vi "Begin.vi"(8 "error in":errorcluster) -> (0 "error out":errorcluster)   [LabVIEW 2017]
doc: "Called before other user functions, this VI is expected to open initial I/O refnums, load in file data, and do all program initialization. Notice that the <B>error out</B> terminal is simply used for data flow. Wiring it to other structures or subVIs ensures that this VI runs first."
uses:
  <vilib>/Rock Robotics/WPI/DriverStation/WPI_DriverStationRobotMode2.ctl
  <vilib>/Rock Robotics/WPI/Joystick/WPI_JoystickDeviceEnum.ctl
  <vilib>/Rock Robotics/WPI/Solenoid/WPI_SolenoidChannel.ctl
  <vilib>/Rock Robotics/SystemInterfaces/DIO/FPGA_DIOChannel.ctl
  <vilib>/Rock Robotics/SystemInterfaces/DIO/FPGA_DIOPWMChannel.ctl
  <vilib>/Rock Robotics/SystemInterfaces/spilib/spi_bus.ctl
  Robot Global Data.vi
  <vilib>/Rock Robotics/Network Tables/NT Write String Array.vi
  <vilib>/Rock Robotics/WPI/Solenoid/WPI_SolenoidOpenDouble.vi
  <vilib>/Rock Robotics/WPI/Ultrasonic/WPI_SonarMB1010DigitalOpen.vi
  <vilib>/Rock Robotics/WPI/Ultrasonic/WPI_SonarMB1010DigRefNum Registry Set.vi
  <vilib>/Rock Robotics/WPI/Switch/WPI_SwitchOpenLimit.vi
  <vilib>/Rock Robotics/WPI/MotorControl/WPI_MotorControlOpen VictorSP.vi
  <vilib>/Rock Robotics/WPI/Gyro/WPI_GyroXRS450_SPI_Open.vi
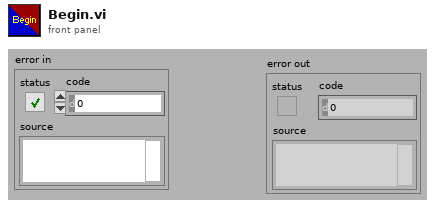
[diagram p1: front panel]
types:
  T1 = typedef "spi_bus.ctl" = enum16{"SPI On-Board, CS0", "SPI On-Board, CS1", "SPI On-Board, CS2", "SPI On-Board, CS3", "SPI MXP", "Invalid"}
  T2 = typedef "FPGA_DIOPWMChannel.ctl" = enum8{"PWM 0", "PWM 1", "PWM 2", "PWM 3", "PWM 4", "PWM 5", "PWM 6", "PWM 7", "PWM 8", "PWM 9", "PWM MXP 0", "PWM MXP 1", "PWM MXP 2", "PWM MXP 3", "PWM MXP 4", "PWM MXP 5", "PWM MXP 6", "PWM MXP 7", "PWM MXP 8", "PWM MXP 9", "Invalid"}
  T3 = typedef "FPGA_DIOChannel.ctl" = enum8{"DIO 0", "DIO 1", "DIO 2", "DIO 3", "DIO 4", "DIO 5", "DIO 6", "DIO 7", "DIO 8", "DIO 9", "DIO MXP 0", "DIO MXP 1", "DIO MXP 2", "DIO MXP 3", "DIO MXP 4", "DIO MXP 5", "DIO MXP 6", "DIO MXP 7", "DIO MXP 8", "DIO MXP 9", "DIO MXP 10", "DIO MXP 11", "DIO MXP 12", "DIO MXP 13", "DIO MXP 14", "DIO MXP 15", "SPI Port CS1", "SPI Port CS2", "SPI Port CS3", "SPI Port MISO", "SPI Port MOSI", "Invalid"}
  T4 = typedef "WPI_SolenoidChannel.ctl" = enum8{"Solenoid 0", "Solenoid 1", "Solenoid 2", "Solenoid 3", "Solenoid 4", "Solenoid 5", "Solenoid 6", "Solenoid 7", "Invalid"}
  T5 = typedef "WPI_JoystickDeviceEnum.ctl" = enum16{"USB 0", "USB 1", "USB 2", "USB 3", "USB 4", "USB 5"}
  T6 = typedef "WPI_DriverStationRobotMode2.ctl" = enum16{"Autonomous Disabled", "Autonomous Enabled", "Teleop Disabled", "Teleop Enabled", "Disconnected", "Finish", "Test Disabled", "Test Enabled", "Emergency Stopped"}
  T7 = typedef "WPI_MotorControlDeviceRef.ctl" = cluster{"DeviceStatus":errorcluster, "Type":T8, "PWM":cluster{"PWM Channel":T2, "DeadBand":T9}, "CAN":cluster{"Device Number":u8, "SetOutput VI Ref":variant, "GetOutput VI Ref":variant, "Enable VI Ref":variant, "Disable VI Ref":variant, "Data":variant}, "Invert":bool, "DIO PWM":cluster{"PWM \"Enable\" Channel":T2, "DIOChannel":T3, "PWM Rate":dbl}}
  T8 = typedef "WPI_MotorControlType.ctl" = enum16{"PWM", "CAN", "DIO PWM"}
  T9 = typedef "WPI_PWMDeadband.ctl" = cluster{"Name":string, "maxPositivePwm":i32, "minPositivePwm":i32, "centerPwm":i32, "maxNegativePwm":i32, "minNegativePwm":i32, "angularRange":u16}
  T10 = typedef "WPI_SwitchDevRef.ctl" = cluster{"DevStatus":errorcluster, "DIO Channel":T3, "CntIndex":T11, "Normally Closed":bool}
  T11 = typedef "FPGA_CounterCtrSystemIndex.ctl" = enum8{"Ctr 0", "Ctr 1", "Ctr 2", "Ctr 3", "Ctr 4", "Ctr 5", "Ctr 6", "Ctr 7", "Invalid"}
  T12 = typedef "WPI_SonarMB1010DigitalDeviceRef.ctl" = cluster{"CounterDevRef":T13, "Scaling factor (s/in)":dbl}
  T13 = typedef "WPI_CounterDevRef.ctl" = cluster{"DevStatus":errorcluster, "CntIndex":T11}
  T14 = typedef "WPI_GyroDevRef.ctl" = cluster{"DevStatus":errorcluster, "Analog Channel":T15, "Gain (VoltsPerDegree/Second)":dbl, "Gyro Type":enum16{"Analog", "XRS450"}, "Handle":i32, "SPI Bus":T1, "Device Found":bool, "Sample Rate":dbl, "Calibrate On Open":bool, "Offset":dbl}
  T15 = typedef "FPGA_AIChannel.ctl" = enum8{"AI 0", "AI 1", "AI 2", "AI 3", "AI MXP 0", "AI MXP 1", "AI MXP 2", "AI MXP 3", "Invalid"}
  T16 = typedef "WPI_SolenoidDevRef.ctl" = cluster{"DevStatus":errorcluster, "Pneumatics Control Module":u8, "Forward Solenoid Channel":T4, "Reverse Solenoid Channel":T4}
  T17 = typedef "WPI_JoystickDevRef.ctl" = cluster{"Device":T5}
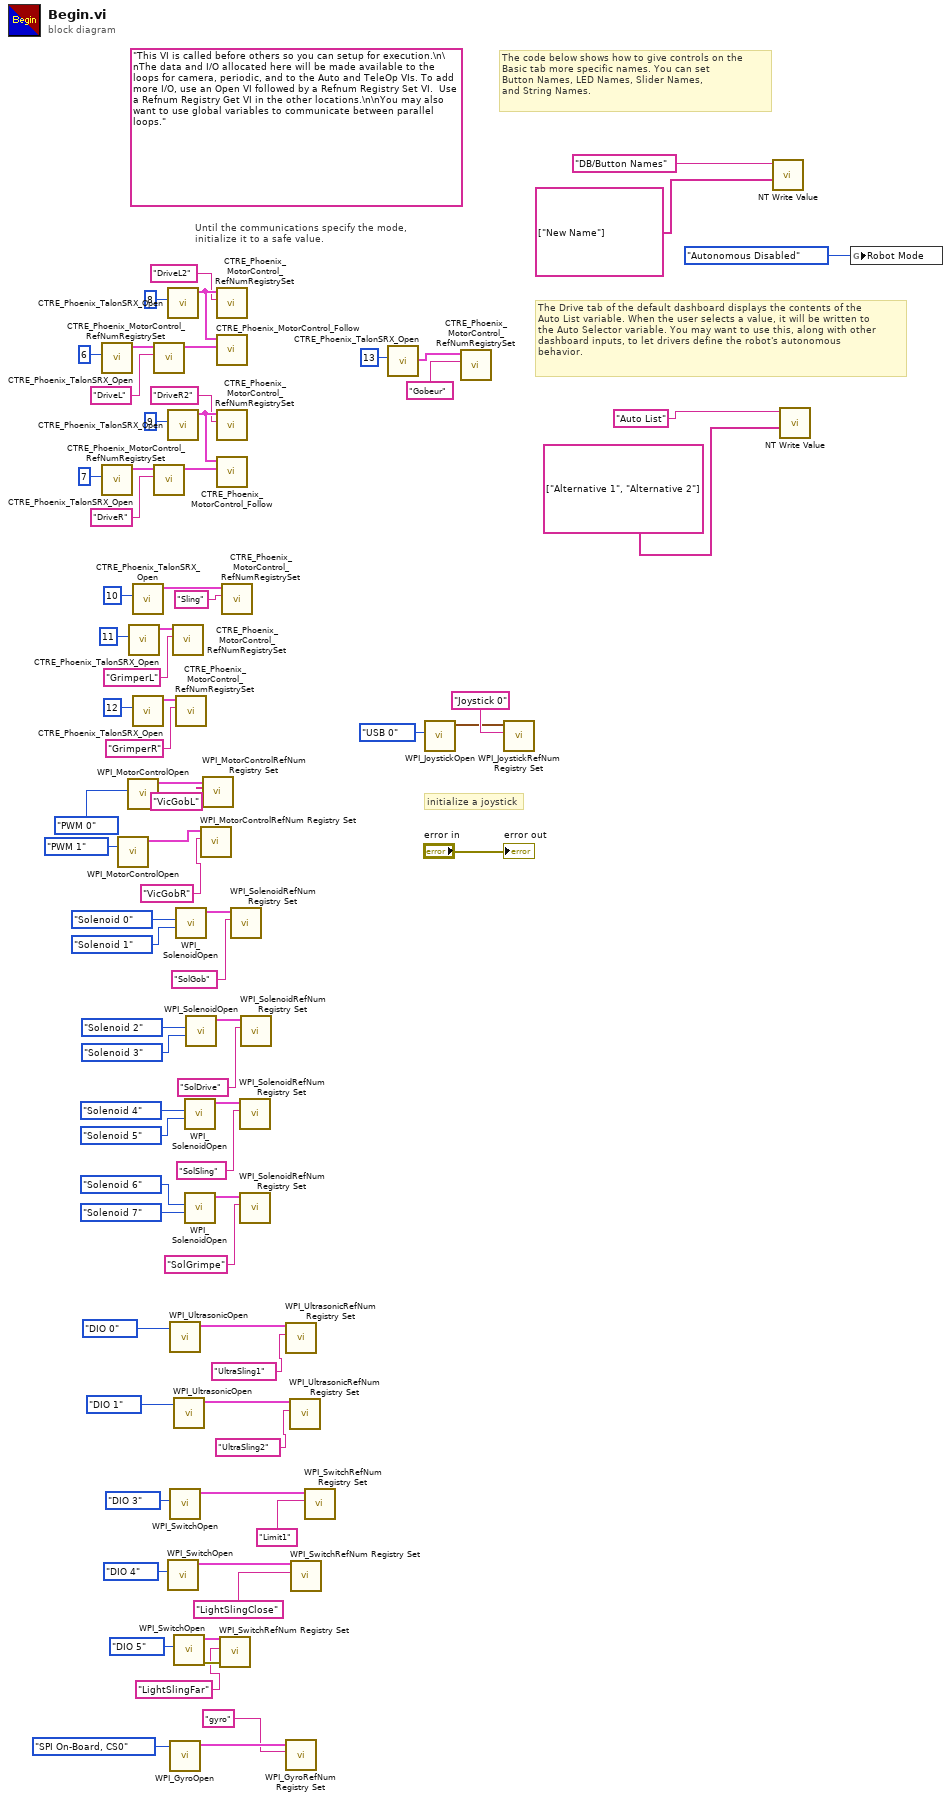
[diagram p0: block diagram]
diagram:
  (unwired) "This VI is called before others so you can setup for execution.\n\nThe data and I/O allocated here will be made available to the loops for camera, periodic, and to the Auto and TeleOp VIs. To add more I/O, use an Open VI followed by a Refnum Registry Set VI.  Use a Refnum Registry Get VI in the other locations.\n\nYou may also want to use global variables to communicate between parallel loops."
  # "The Drive tab of the default dashboard displays the contents of the\nAuto List variable. When the user selects a value, it will be written to\nthe Auto Selector variable. You may want to use this, along with other\ndashboard inputs, to let drivers define the robot's autonomous\nbehavior."
  # "The code below shows how to give controls on the\nBasic tab more specific names. You can set\nButton Names, LED Names, Slider Names,\nand String Names."
  # "initialize a joystick"
  # "Until the communications specify the mode,\ninitialize it to a safe value."
  n1 = call "CTRE_Phoenix_TalonSRX_Open.vi"("Device Number"=u8 6) -> ("CAN Talon SRX Ref"=w67:T7)  [unwired: 9 in, 1 out]
  n2 = call "CTRE_Phoenix_TalonSRX_Open.vi"("Device Number"=u8 7) -> ("CAN Talon SRX Ref"=w66:T7)  [unwired: 9 in, 1 out]
  n3 = call-poly <vilib>:"WPI_MotorControlOpen.vi"("PWM Channel"=FPGA_DIOPWMChannel."PWM 1") -> ("MotorControlDeviceRef"=w21:T7)  [unwired: 9 in, 1 out]
  n4 = call-poly <vilib>:"WPI_MotorControlOpen.vi"("PWM Channel"=FPGA_DIOPWMChannel."PWM 0") -> ("MotorControlDeviceRef"=w20:T7)  [unwired: 9 in, 1 out]
  n5 = call "CTRE_Phoenix_TalonSRX_Open.vi"("Device Number"=u8 11) -> ("CAN Talon SRX Ref"=w64:T7)  [unwired: 9 in, 1 out]
  n6 = call "CTRE_Phoenix_TalonSRX_Open.vi"("Device Number"=u8 10) -> ("CAN Talon SRX Ref"=w65:T7)  [unwired: 9 in, 1 out]
  n7 = call "CTRE_Phoenix_TalonSRX_Open.vi"("Device Number"=u8 12) -> ("CAN Talon SRX Ref"=w63:T7)  [unwired: 9 in, 1 out]
  n8 = call "CTRE_Phoenix_MotorControl_RefNumRegistrySet.vi"("refnum name"="DriveL", "PhoenixMotorControlDevRef"=w67) -> ("PhoenixMotorControlDevRef"=w9:T7)  [unwired: 8 in, 1 out]
  n9 = call "CTRE_Phoenix_MotorControl_RefNumRegistrySet.vi"("refnum name"="DriveR", "PhoenixMotorControlDevRef"=w66) -> ("PhoenixMotorControlDevRef"=w8:T7)  [unwired: 8 in, 1 out]
  n10 = call "CTRE_Phoenix_TalonSRX_Open.vi"("Device Number"=u8 8) -> ("CAN Talon SRX Ref"=w4:T7)  [unwired: 9 in, 1 out]
  n11 = call "CTRE_Phoenix_TalonSRX_Open.vi"("Device Number"=u8 9) -> ("CAN Talon SRX Ref"=w3:T7)  [unwired: 9 in, 1 out]
  n12 = call-poly <vilib>:"WPI_SwitchOpen.vi"("DIO Channel"=FPGA_DIOChannel."DIO 4") -> ("SwitchDevRef"=w26:T10)  [unwired: 9 in, 1 out]
  n13 = call-poly <vilib>:"WPI_UltrasonicOpen.vi"("DIO Channel"=FPGA_DIOChannel."DIO 0") -> ("SonarMB1010DigitalDevRef"=w33:T12)  [unwired: 9 in, 1 out]
  n14 = call-poly <vilib>:"WPI_SwitchOpen.vi"("DIO Channel"=FPGA_DIOChannel."DIO 3") -> ("SwitchDevRef"=w25:T10)  [unwired: 9 in, 1 out]
  n15 = call-poly <vilib>:"WPI_GyroOpen.vi"("SPI Bus"=spi_bus."SPI On-Board, CS0") -> ("GyroDevRef"=w6:T14)  [unwired: 8 in, 2 out]
  n16 = call "CTRE_Phoenix_MotorControl_RefNumRegistrySet.vi"("refnum name"="GrimperL", "PhoenixMotorControlDevRef"=w64) -> ()  [unwired: 8 in, 2 out]
  n17 = call-poly <vilib>:"WPI_UltrasonicOpen.vi"("DIO Channel"=FPGA_DIOChannel."DIO 1") -> ("SonarMB1010DigitalDevRef"=w30:T12)  [unwired: 9 in, 1 out]
  n18 = call-poly <vilib>:"WPI_SwitchOpen.vi"("DIO Channel"=FPGA_DIOChannel."DIO 5") -> ("error out"=w28:errorcluster, "SwitchDevRef"=w27:T10)  [unwired: 9 in]
  n19 = call "CTRE_Phoenix_MotorControl_RefNumRegistrySet.vi"("refnum name"="GrimperR", "PhoenixMotorControlDevRef"=w63) -> ()  [unwired: 8 in, 2 out]
  n20 = call-poly <vilib>:"WPI_SolenoidOpen.vi"("Reverse Solenoid Channel"=WPI_SolenoidChannel."Solenoid 1", "Forward Solenoid Channel"=WPI_SolenoidChannel."Solenoid 0") -> ("SolenoidDevRef"=w50:T16)  [unwired: 8 in, 1 out]
  n21 = call-poly <vilib>:"WPI_SolenoidOpen.vi"("Reverse Solenoid Channel"=WPI_SolenoidChannel."Solenoid 5", "Forward Solenoid Channel"=WPI_SolenoidChannel."Solenoid 4") -> ("SolenoidDevRef"=w48:T16)  [unwired: 8 in, 1 out]
  n22 = call-poly <vilib>:"WPI_SolenoidOpen.vi"("Reverse Solenoid Channel"=WPI_SolenoidChannel."Solenoid 7", "Forward Solenoid Channel"=WPI_SolenoidChannel."Solenoid 6") -> ("SolenoidDevRef"=w47:T16)  [unwired: 8 in, 1 out]
  n23 = call-poly <vilib>:"WPI_SolenoidOpen.vi"("Reverse Solenoid Channel"=WPI_SolenoidChannel."Solenoid 3", "Forward Solenoid Channel"=WPI_SolenoidChannel."Solenoid 2") -> ("SolenoidDevRef"=w49:T16)  [unwired: 8 in, 1 out]
  n24 = call <vilib>:"WPI_MotorControlRefNum Registry Set.vi"("refnum name"="VicGobR", "MotorControlDevRef"=w21) -> ()  [unwired: 8 in, 2 out]
  n25 = call <vilib>:"WPI_MotorControlRefNum Registry Set.vi"("refnum name"="VicGobL", "MotorControlDevRef"=w20) -> ()  [unwired: 8 in, 2 out]
  n26 = call "CTRE_Phoenix_MotorControl_RefNumRegistrySet.vi"("refnum name"="DriveL2", "PhoenixMotorControlDevRef"=w4) -> ()  [unwired: 8 in, 2 out]
  n27 = call "CTRE_Phoenix_MotorControl_Follow.vi"("Master Controller to Follow"=w9, "PhoenixMotorControlDevRef"=w4) -> ()  [unwired: 8 in, 2 out]
  n28 = call "CTRE_Phoenix_MotorControl_RefNumRegistrySet.vi"("refnum name"="DriveR2", "PhoenixMotorControlDevRef"=w3) -> ()  [unwired: 8 in, 2 out]
  n29 = call "CTRE_Phoenix_MotorControl_Follow.vi"("Master Controller to Follow"=w8, "PhoenixMotorControlDevRef"=w3) -> ()  [unwired: 8 in, 2 out]
  n30 = call <vilib>:"WPI_SwitchRefNum Registry Set.vi"("error in (no error)"=w28, "refnum name"="LightSlingFar", "SwitchDevRef"=w27) -> ()  [unwired: 7 in, 2 out]
  n31 = call "CTRE_Phoenix_MotorControl_RefNumRegistrySet.vi"("refnum name"="Sling", "PhoenixMotorControlDevRef"=w65) -> ()  [unwired: 8 in, 2 out]
  n32 = call <vilib>:"WPI_SolenoidRefNum Registry Set.vi"("refnum name"="SolGob", "SolenoidDevRef"=w50) -> ()  [unwired: 8 in, 2 out]
  n33 = call <vilib>:"WPI_SolenoidRefNum Registry Set.vi"("refnum name"="SolSling", "SolenoidDevRef"=w48) -> ()  [unwired: 8 in, 2 out]
  n34 = call <vilib>:"WPI_SolenoidRefNum Registry Set.vi"("refnum name"="SolGrimpe", "SolenoidDevRef"=w47) -> ()  [unwired: 8 in, 2 out]
  n35 = call <vilib>:"WPI_SolenoidRefNum Registry Set.vi"("refnum name"="SolDrive", "SolenoidDevRef"=w49) -> ()  [unwired: 8 in, 2 out]
  n36 = call-poly <vilib>:"WPI_UltrasonicRefNum Registry Set.vi"("refnum name"="UltraSling1", "SonarMB1010DigitalDevRef"=w33) -> ()  [unwired: 8 in, 2 out]
  n37 = call <vilib>:"WPI_GyroRefNum Registry Set.vi"("refnum name"="gyro", "GyroDevRef"=w6) -> ()  [unwired: 8 in, 2 out]
  n38 = call-poly <vilib>:"WPI_UltrasonicRefNum Registry Set.vi"("refnum name"="UltraSling2", "SonarMB1010DigitalDevRef"=w30) -> ()  [unwired: 8 in, 2 out]
  n39 = call <vilib>:"WPI_SwitchRefNum Registry Set.vi"("refnum name"="LightSlingClose", "SwitchDevRef"=w26) -> ()  [unwired: 8 in, 2 out]
  n40 = call <vilib>:"WPI_SwitchRefNum Registry Set.vi"("refnum name"="Limit1", "SwitchDevRef"=w25) -> ()  [unwired: 8 in, 2 out]
  n41 = call "CTRE_Phoenix_TalonSRX_Open.vi"("Device Number"=u8 13) -> ("CAN Talon SRX Ref"=w12:T7)  [unwired: 9 in, 1 out]
  n42 = call <vilib>:"WPI_JoystickOpen.vi"("JoystickDevice"=WPI_JoystickDeviceEnum."USB 0") -> ("JoystickDevRef"=w74:T17)  [unwired: 10 in]
  n43 = call "CTRE_Phoenix_MotorControl_RefNumRegistrySet.vi"("refnum name"="Gobeur", "PhoenixMotorControlDevRef"=w12) -> ()  [unwired: 8 in, 2 out]
  n44 = call <vilib>:"WPI_JoystickRefNum Registry Set.vi"("refnum name"="Joystick 0", "JoystickDevRef"=w74) -> ()  [unwired: 8 in, 2 out]
  n45 = call-poly <vilib>:"NT Write Value.vi"("String Array"=string[] ["New Name"], "Name"="DB/Button Names") -> ()  [unwired: 9 in, 1 out]
  n46 = call-poly <vilib>:"NT Write Value.vi"("String Array"=string[] ["Alternative 1", "Alternative 2"], "Name"="Auto List") -> ()  [unwired: 9 in, 1 out]
  n47 = global write "Robot Global Data.vi" "Robot Mode"(WPI_DriverStationRobotMode2."Autonomous Disabled" ("Robot Mode")) -> ()
  "error out" <- "error in"
